vi "Configure Measurement Averaging.vi"(0 "VISA resource name":refnum<visa-resource-name>, 1 "Averaging Mode (0: Exponential)":u16(ring) items=["Exponential", "Repeat"], 5 "Measurement Type (0: Adjacent Channel Power)":u16(ring) items=["Adjacent Channel Power"=0, "Burst Power"=1, "Channel Power"=2, "Harmonics Distortion"=3, "Intermod"=4, "Multi-Carrier Power"=5, "Occupied Bandwidth"=6, "Spectrum Emissions Mask"=8, "Spurious Emissions"=9], 7 "Enable Averaging (Enable)":bool=TRUE, 9 "Average Number (10)":i32=10, 11 "error in (no error)":errorcluster) -> (4 "VISA resource name out":refnum<visa-resource-name>, 15 "error out":errorcluster)   [LabVIEW 2014, in "Agilent ESA PSA Series.lvlib"]
doc: "Configures measurement averaging."
uses:
  Agilent ESA PSA Series.lvlib
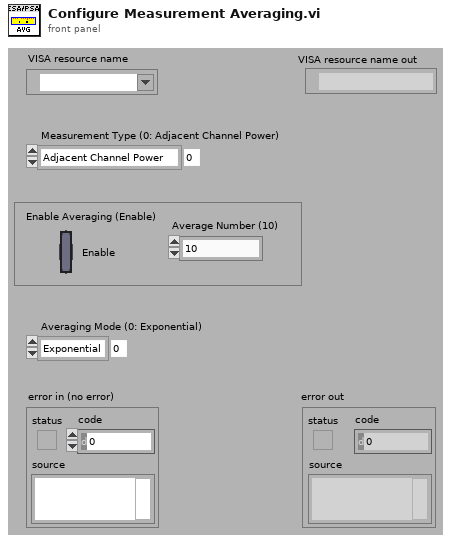
[diagram p1: front panel]
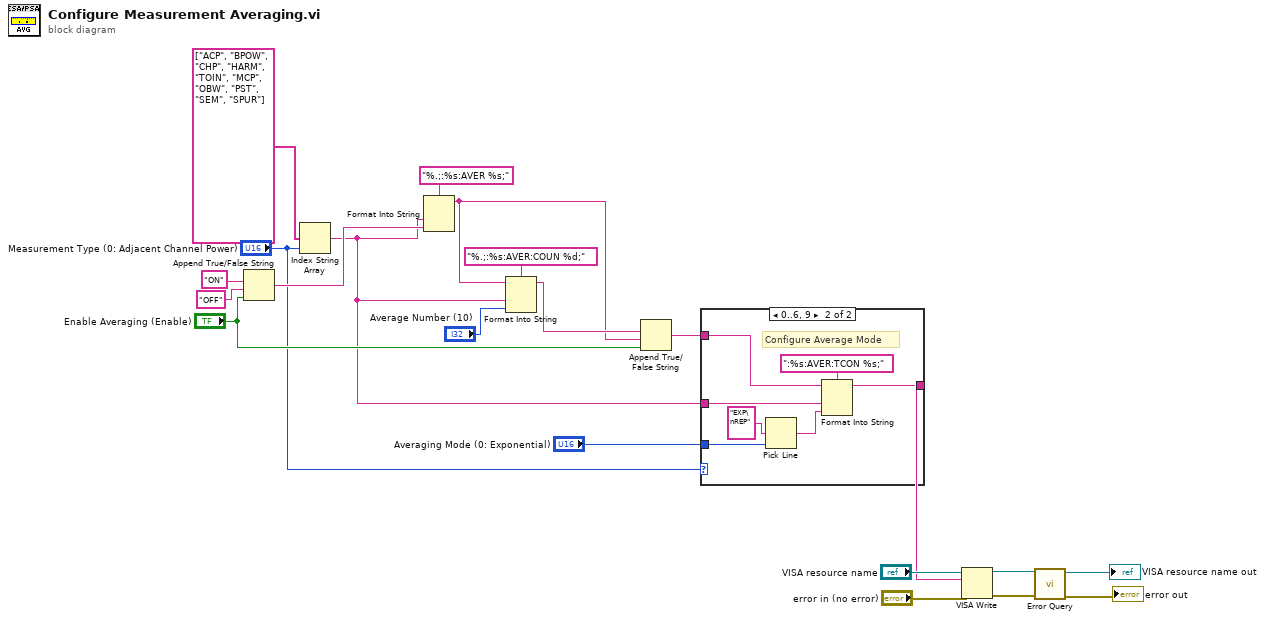
[diagram p0: block diagram]
diagram:
  n1 = Append True/False String(1:"Enable Averaging (Enable)", 2:"OFF" ("true string"), 3:"ON" ("true string")) -> (0:w15:string)  [unwired: 1 in]
  n2 = Index String Array(1:"Measurement Type (0: Adjacent Channel Power)", 2:string[] ["ACP", "BPOW", "CHP", "HARM", "TOIN", "MCP", "OBW", "PST", "SEM", "SPUR"]) -> (0:w5:string)  [unwired: 1 in]
  n3 = Format Into String(format string="%.;:%s:AVER %s;", w5, w15) -> (resulting string=w12:string)  [unwired: 2 in, 1 out]
  n4 = Format Into String(format string="%.;:%s:AVER:COUN %d;", initial string=w12, w5, "Average Number (10)") -> (resulting string=w13:string)  [unwired: 1 in, 1 out]
  n5 = Append True/False String(1:"Enable Averaging (Enable)", 2:w12, 3:w13) -> (0:w6:string)  [unwired: 1 in]
  n6 = case shown="0..6, 9" "Measurement Type (0: Adjacent Channel Power)" {
    tunnel: "Averaging Mode (0: Exponential)" -> [_ w28]
    tunnel: w6 -> [w22 w25]
    tunnel: [w22 w24] -> w1
    tunnel: w5 -> [_ w23]
    frame 8, Default {
      # "Spectrum Emission Mask doesn't\nsupport Average Mode."
    }
    frame 0..6, 9 {
      # "Configure Average Mode"
      n7 = Pick Line(multi-line string="EXP\nREP", line index=w28) -> (output string=w26:string)  [unwired: 1 in]
      n8 = Format Into String(format string=":%s:AVER:TCON %s;", initial string=w25, w23, w26) -> (resulting string=w24:string)  [unwired: 1 in, 1 out]
    }
  }
  n9 = VISA Write(VISA resource name="VISA resource name", write buffer=w1, error in (no error)="error in (no error)") -> (VISA resource name out=w4:refnum<visa-resource-name>, error out=w3:errorcluster)  [unwired: 1 out]
  n10 = call "Error Query.vi"("error in (no error)"=w3, "VISA resource name"=w4) -> ("error out"=→"error out":errorcluster, "VISA resource name out"=→"VISA resource name out":refnum<visa-resource-name>)  [unwired: 6 in, 2 out]
